vi "Init.vi"(8 "error in (no error)":errorcluster, 10 "VectoService":refnum<class "VectoInfo.lvclass">) -> (0 "error out":errorcluster, 3 "HTTPStatsHandler out":refnum<class "HTTPStatsHandler.lvclass">)   [LabVIEW 2020, in "Vecto.lvlib" / "HTTPStatsHandler.lvclass"]
uses:
  HTTPStatsHandler.lvclass
  VectoService/VectoInfo.lvclass
  HTTPStatsHandler.lvclass/HTTPStatsHandler.ctl
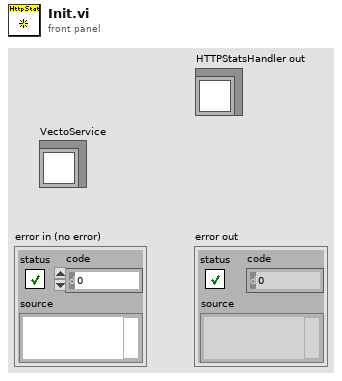
[diagram p1: front panel]
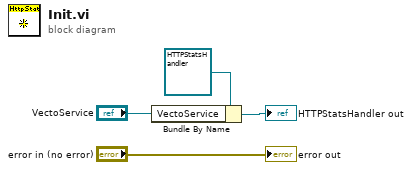
[diagram p0: block diagram]
diagram:
  n1 = Bundle By Name(cluster=refnum<class "HTTPStatsHandler.lvclass"> refnum ("HTTPStatsHandler in"), "VectoService"="VectoService") -> (→"HTTPStatsHandler out":refnum<class "HTTPStatsHandler.lvclass">)
  "error out" <- "error in (no error)"
